vi "DAC Configure.vi"(8 "error in":errorcluster, 11 "DAC LN2 Temp in":refnum<class "DAC LN2 Temp.lvclass">) -> (0 "error out":errorcluster, 3 "DAC LN2 Temp out":refnum<class "DAC LN2 Temp.lvclass">)   [LabVIEW 2019, in "DAC.lvlib" / "DAC LN2 Temp.lvclass"]
uses:
  DAC LN2 Temp.lvclass
  C:/Users/krio/Documents/LV_Projects/test-stand/App/DAC/DAC.lvclass
  DAC.lvclass/DAC.ctl
  DAC LN2 Temp.lvclass/DAC LN2 Temp.ctl
  <vilib>/DAQmx/create/channels.llb/DAQmx Create Channel (AI-Temperature-RTD).vi
  DAC.lvclass
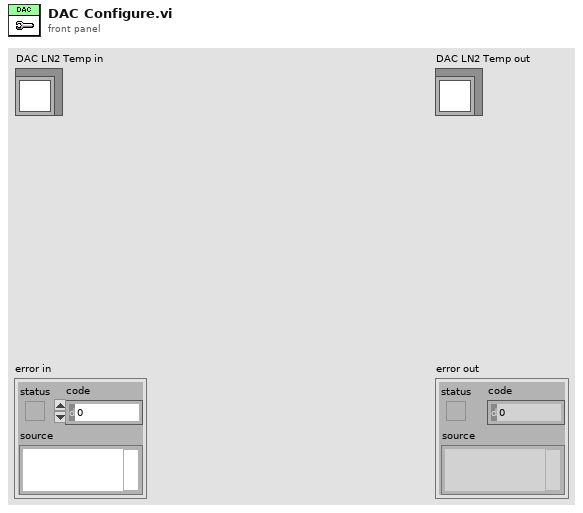
[diagram p1: front panel]
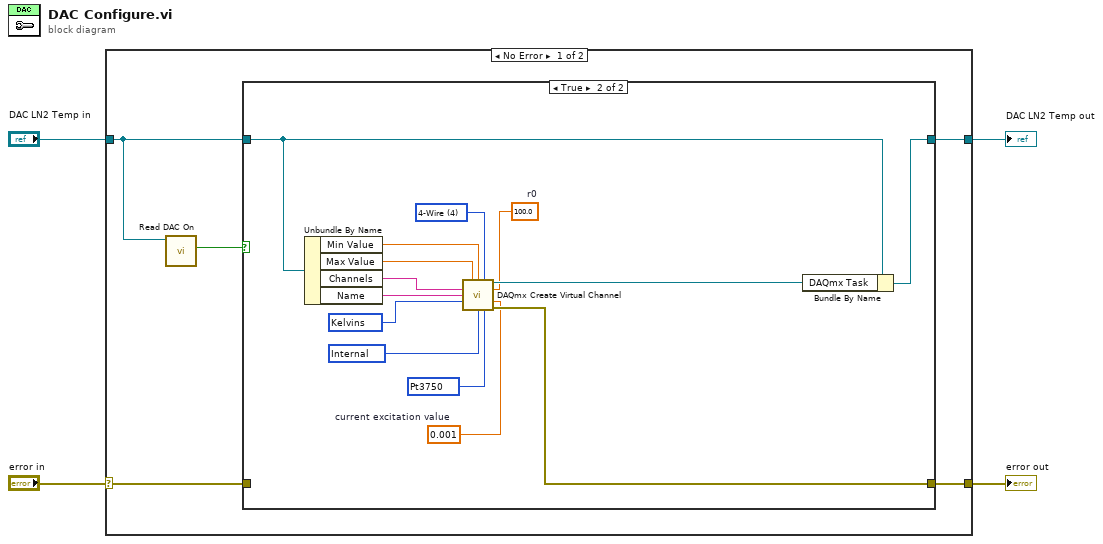
[diagram p0: block diagram]
diagram:
  n1 = case shown="No Error" "error in" {
    selector: "error in" -> [w6 w27]
    tunnel: [w5 w27] -> w4
    tunnel: [w7 w26] -> w3
    tunnel: "DAC LN2 Temp in" -> [w9 w26]
    frame No Error {
      n2 = call "Read DAC On.vi"("DAC in"=w9) -> ("DAC On"=w8:bool)  [unwired: 8 in, 2 out]
      n3 = case shown="True" w8 {
        tunnel: w9 -> [w11 w24]
        tunnel: [w11 w23] -> w7
        tunnel: w6 -> [w10 _]
        tunnel: [w10 w18] -> w5
        frame False {
          # "Temperature measurement is off."
        }
        frame True {
          w12 = 0.001  # current excitation value
          w13 = 12481 items=["Pt3750"=12481, "Pt3851"=10071, "Pt3911"=12482, "Pt3916"=10069, "Pt3920"=10053, "Pt3928"=12483, "Custom"=10137] ("rtd type")
          w14 = 10200 items=["Internal"=10200, "External"=10167, "None"=10230] ("current excitation source")
          w15 = 100.0  # r0
          w16 = 4 items=["2-Wire"=2, "3-Wire"=3, "4-Wire"=4] ("resistance configuration")
          w17 = 10325 items=["Deg C"=10143, "Deg F"=10144, "Kelvins"=10325, "Deg R"=10145, "From Custom Scale"=10065] ("units")
          # "Temperature measurement is on."
          n4 = Unbundle By Name(w24) -> ("Min Value"=w20:dbl, "Max Value"=w25:dbl, "Channels"=w22:string, "Name"=w21:string)
          n5 = call-poly <vilib>:"DAQmx Create Virtual Channel.vi"("maximum value"=w25, "minimum value"=w20, "resistance configuration"=w16, "physical channels"=w22, "r0"=w15, "name to assign"=w21, "units"=w17, "current excitation value"=w12, "current excitation source"=w14, "rtd type"=w13) -> ("task out"=w19:refnum<k21>, "error out"=w18:errorcluster)  [unwired: 4 in]
          n6 = Bundle By Name(cluster=w24, "DAQmx Task"=w19) -> (w23:refnum<class "DAC LN2 Temp.lvclass">)
        }
      }
    }
    frame Error {
    }
  }
  "error out" <- w4
  "DAC LN2 Temp out" <- w3
